vi "CloseDevice.vi"(4 "Error In":errorcluster) -> (0 "Error Out":errorcluster)   [LabVIEW 2020]
doc: "Dummy VI which simulate subVI to close some device."
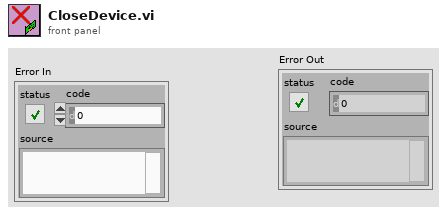
[diagram p1: front panel]
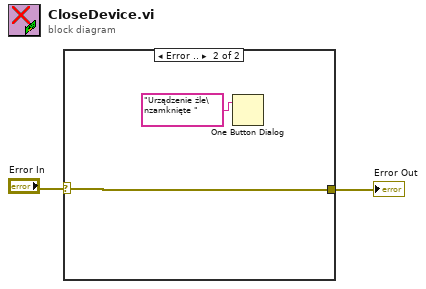
[diagram p0: block diagram]
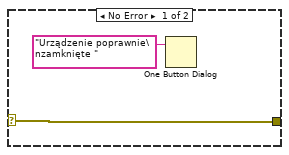
[diagram p2: hidden frame]
diagram:
  n1 = case shown="Error .." "Error In" {
    selector: "Error In" -> [w4 w6]
    tunnel: [w4 w6] -> w1
    frame No Error {
      n2 = One Button Dialog(message="Urządzenie poprawnie\nzamknięte ") -> ()  [unwired: 1 in, 1 out]
    }
    frame Error {
      n3 = One Button Dialog(message="Urządzenie źle\nzamknięte ") -> ()  [unwired: 1 in, 1 out]
    }
  }
  "Error Out" <- w1
